vi "Object Results.vi"(0 "Object Start/Stop/Sum in":i32[][](array[numeric]), 7 "Offset rows,cols":i32[](array[numeric]), 9 "Image rows,cols":i32[](array[numeric])) -> (11 "Pixels Up":i32, 13 "Pixels Rt":i32, 14 "Object Start/Stop/Sum out":i32[][](array[numeric]), 19 "Pixel Sum":i32)   [LabVIEW 2016]
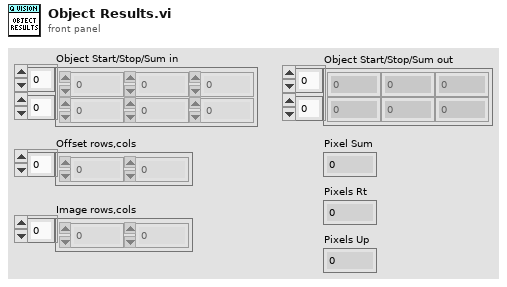
[diagram p1: front panel]
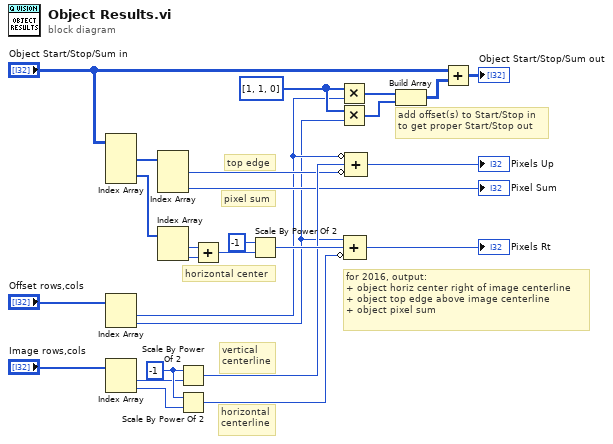
[diagram p0: block diagram]
diagram:
  w5 = i32[] [1, 1, 0]
  w14 = i16 -1 ("n")
  # "add offset(s) to Start/Stop in\nto get proper Start/Stop out"
  # "for 2016, output:\n+ object horiz center right of image centerline\n+ object top edge above image centerline\n+ object pixel sum"
  # "pixel sum"
  # "horizontal\ncenterline"
  # "vertical\ncenterline"
  # "top edge"
  # "horizontal center"
  n1 = Index Array(array="Object Start/Stop/Sum in") -> (element #1=w24:i32[], element #2=w25:i32[])  [unwired: 4 in]
  n2 = Index Array(array="Offset rows,cols") -> (element #1=w2:i32, element #2=w1:i32)  [unwired: 2 in]
  n3 = Index Array(array="Image rows,cols") -> (element #1=w12:i32, element #2=w13:i32)  [unwired: 2 in]
  n4 = Index Array(array=w24) -> (element #1=w11:i32, element #3=→"Pixel Sum":i32)  [unwired: 3 in, 1 out]
  n5 = Index Array(array=w25) -> (element #1=w22:i32, element #2=w23:i32)  [unwired: 2 in]
  n6 = Scale By Power Of 2(n=w14, x=w12) -> (x*2^n=w18:i32)
  n7 = Scale By Power Of 2(n=w14, x=w13) -> (x*2^n=w17:i32)
  n8 = Add(x=w22, y=w23) -> (x+y=w16:i32)
  n9 = Scale By Power Of 2(n=i16 -1, x=w16) -> (x*2^n=w21:i32)
  n10 = Multiply(x=w5, y=w2) -> (x*y=w4:i32[])
  n11 = Multiply(x=w5, y=w1) -> (x*y=w3:i32[])
  n12 = Compound Arithmetic op=ADD(w1, w21, invert w17) -> (→"Pixels Rt":i32)
  n13 = Compound Arithmetic op=ADD(invert w2, w18, invert w11) -> (→"Pixels Up":i32)
  n14 = Build Array(w4, w3) -> (w9:i32[][])
  n15 = Add(x="Object Start/Stop/Sum in", y=w9) -> (x+y=→"Object Start/Stop/Sum out":i32[][])
